vi "SRV_PM_Create Packet.vi"(0 "Command Type":string, 1 "Sender (0x01 PC)":u8=1 format="%.0x", 7 "Data String":string, 11 "error in (no error)":errorcluster) -> (10 "Packet":u8[](array[numeric]) format="%.0x", 15 "error out":errorcluster)   [LabVIEW 2009]
panel:
  out "Command Type":u8 format="%.0x"
  out "Data":u8[](array[numeric]) format="%.0x"
  # "Sync"
  # "Command Type"
  # "Sender"
  # "TimeStamp"
  # "Data Length"
  # "Data\n.\n\nLast 2 Bytes are CRC-16"
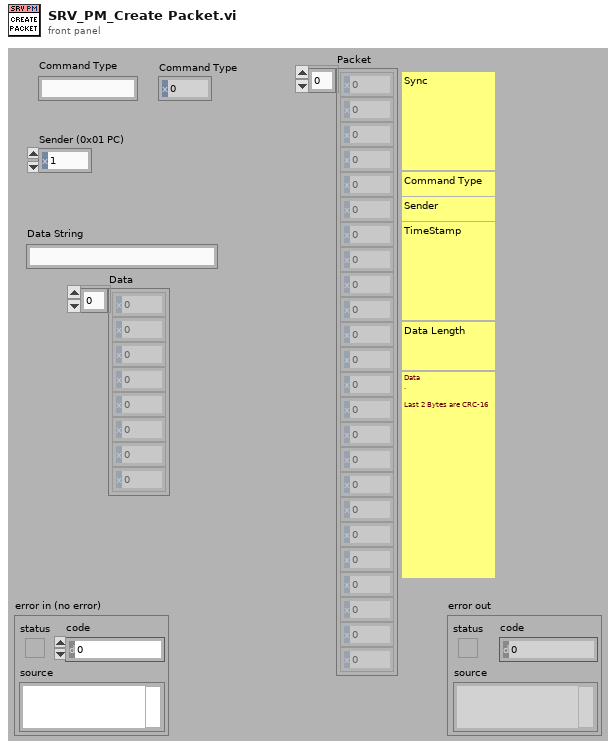
[diagram p1: front panel]
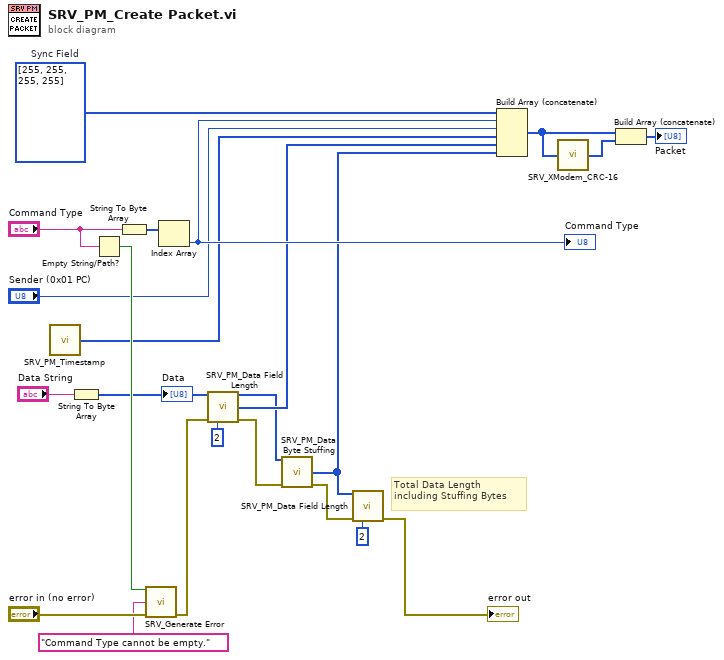
[diagram p0: block diagram]
diagram:
  w23 = u8[] [255, 255, 255, 255]  # Sync Field
  # "Total Data Length including Stuffing Bytes"
  n1 = call "SRV_PM_Timestamp.vi"() -> ("Timestamp bytes"=w15:u8[])  [unwired: 14 in, 1 out]
  n2 = String To Byte Array(string="Data String") -> (unsigned byte array=w2:u8[])
  "Data" <- w2
  n3 = Empty String/Path?(string/path="Command Type") -> (empty?=w18:bool)
  n4 = String To Byte Array(string="Command Type") -> (unsigned byte array=w22:u8[])
  n5 = call "SRV_Generate Error.vi"("status (T)"=w18, "Message"="Command Type cannot be empty.", "error in (no error)"="error in (no error)") -> ("error out"=w13:errorcluster)  [unwired: 12 in]
  n6 = Index Array(array=w22) -> (element=w21:u8)  [unwired: 1 in]
  "Command Type" <- w21
  n7 = call "SRV_PM_Data Field Length.vi"("Data"=w2, "error in (no error)"=w13, "Data Field Length Number of Bytes (2)"=2) -> ("Data dup"=w11:u8[], "Data Field Length Bytes"=w14:u8[], "error out"=w10:errorcluster)  [unwired: 10 in]
  n8 = call "SRV_PM_Data Byte Stuffing.vi"("Data"=w11, "error in (no error)"=w10) -> ("Stuffed Data"=w8:u8[], "error out"=w7:errorcluster)  [unwired: 11 in, 1 out]
  n9 = call "SRV_PM_Data Field Length.vi"("Data"=w8, "error in (no error)"=w7, "Data Field Length Number of Bytes (2)"=2) -> ("error out"=→"error out":errorcluster)  [unwired: 10 in, 2 out]
  n10 = Build Array (concatenate)(w23, w21, "Sender (0x01 PC)", w15, w14, w8) -> (w4:u8[])
  n11 = call "SRV_XModem_CRC-16.vi"("Array"=w4) -> ("16-bit CRC Array"=w3:u8[])  [unwired: 14 in]
  n12 = Build Array (concatenate)(w4, w3) -> (→"Packet":u8[])
